vi "Convert DAQmx to DAQ cal.vi"(11 "Calibration in":T1(array[cluster])) -> (3 "Array":T2[](array[typedef]) {"DevTemp" format="%.1f"; "SelfCal.LastTemp" format="%.1f"; "SelfCal.LastDate/Time" format="%<%I:%M %p %m/%d/%Y>T"})   [LabVIEW 2019, in "Instrument.Lockin.lvlib" / "Instrument.DAQ.lvclass"]
uses:
  Instrument.DAQ.lvclass
  Typedefs/DAQ.Calibration--Cluster.ctl
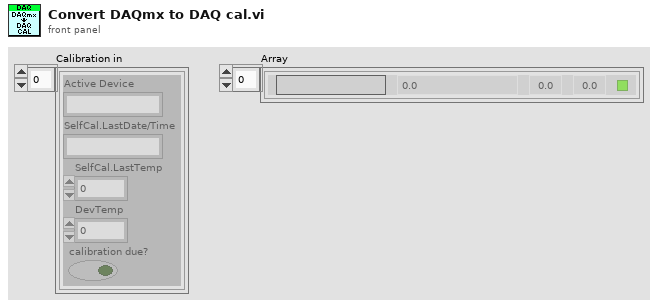
[diagram p1: front panel]
types:
  T1 = cluster{"Active Device":string, "SelfCal.LastDate/Time":string, "SelfCal.LastTemp":dbl, "DevTemp":dbl, "calibration due?":bool}[]
  T2 = typedef "Instrument.Lockin.lvlib/Instrument.DAQ.lvclass/DAQ.Calibration--Cluster.ctl" = cluster{"Active Device":string, "SelfCal.LastDate/Time":dbl, "SelfCal.LastTemp":dbl, "DevTemp":dbl, "calibration due?":bool}
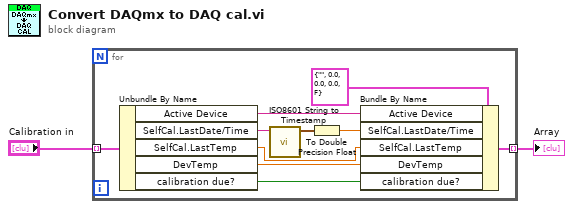
[diagram p0: block diagram]
diagram:
  n1 = for {
    tunnel: "Calibration in" -> [w12] mode=indexing
    tunnel: [w10] -> w2 mode=indexing
    n2 = Unbundle By Name(w12) -> ("Active Device"=w6:string, "SelfCal.LastDate/Time"=w9:string, "SelfCal.LastTemp"=w3:dbl, "DevTemp"=w4:dbl, "calibration due?"=w5:bool)
    n3 = call <vilib>:"ISO8601 String to Timestamp.vi"("ISO8601 String"=w9) -> ("Timestamp"=w8:timestamp)  [unwired: 8 in, 2 out]
    n4 = To Double Precision Float(number=w8) -> (double precision float=w7:dbl)
    n5 = Bundle By Name(cluster=T2 {"Active Device"="", "SelfCal.LastDate/Time"=0.0, "SelfCal.LastTemp"=0.0, "DevTemp"=0.0, "calibration due?"=FALSE} ("Calibration"), "Active Device"=w6, "SelfCal.LastDate/Time"=w7, "SelfCal.LastTemp"=w3, "DevTemp"=w4, "calibration due?"=w5) -> (w10:T2)
  }
  "Array" <- w2
